vi "DeployImage_SC.vi"(8 "error in (no error)":errorcluster, 11 "SysCfgDeployRequest":T1) -> (0 "error out":errorcluster)   [LabVIEW 2016]
uses:
  <vilib>/addons/InsightCM/MessageBus/MessageLibrary/SysCfgDeployer/controls/SysCfgDeployPackageRequestBody.ctl
  <vilib>/nisyscfg/Network Settings Image.ctl
  <vilib>/nisyscfg/Set System Image (File).vi
  <vilib>/nisyscfg/Close (System).vi
  <vilib>/nisyscfg/nisyscfg.lvlib
panel:
  in  "Password":string
  in  "User Name":string="admin"
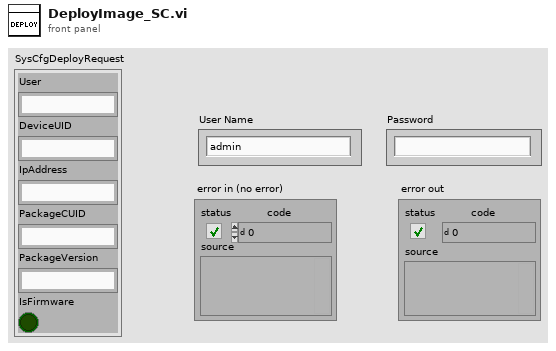
[diagram p1: front panel]
types:
  T1 = typedef "SysCfgDeployPackageRequestBody.ctl" = cluster{"User":string, "DeviceUID":string, "IpAddress":string, "PackageCUID":string, "PackageVersion":string, "IsFirmware":bool}
  T2 = typedef "nisyscfg.lvlib/Network Settings Image.ctl" = u32
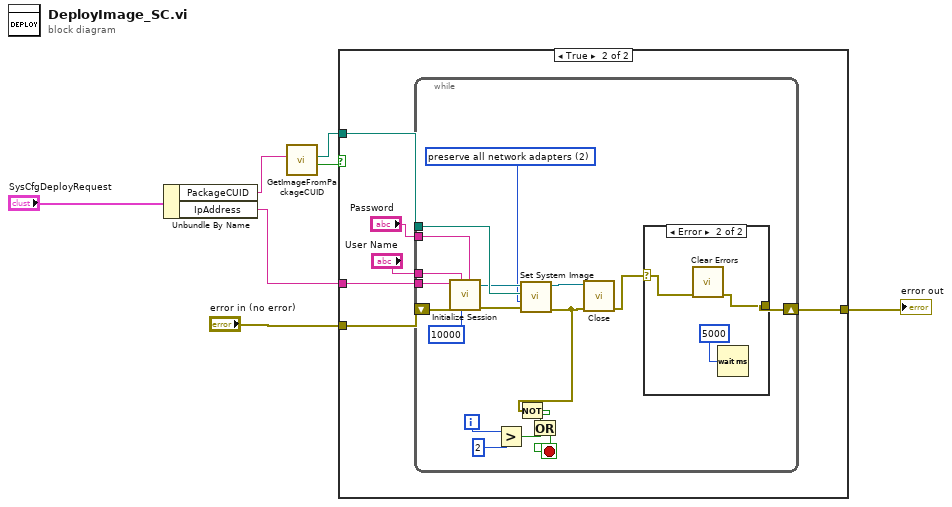
[diagram p0: block diagram]
diagram:
  n1 = Unbundle By Name("SysCfgDeployRequest") -> ("PackageCUID"=w1:string, "IpAddress"=w4:string)
  n2 = call "GetImageFromPackageCUID.vi"("PackageCUID"=w1) -> ("Found"=w2:bool, "path"=w3:path)  [unwired: 9 in]
  n3 = case shown="True" w2 {
    tunnel: "error in (no error)" -> [w8 w14]
    tunnel: [w8 w13] -> w6
    tunnel: w4 -> [_ w12]
    tunnel: w3 -> [_ w9]
    frame False {
    }
    frame True {
      n4 = while {
        tunnel: w9 -> [w32]
        shift-right: [w19] -> w13
        shift-left: w14 -> [w22]
        tunnel: "Password" -> [w24]
        tunnel: "User Name" -> [w23]
        tunnel: w12 -> [w17]
        i -> [w29]
        stop <- w31 stop-if-true
        w16 = T2 2 items=["reset all network adapters", "preserve primary, reset others", "preserve all network adapters", "preserve primary, apply others", "apply primary, reset others", "apply primary, preserve others", "apply all network adapters"] ("Network Settings (preserve primary adapter, apply others)")
        n5 = call <vilib>:"Initialize Session.vi"("Password"=w24, "Connect Timeout (4000 ms)"=u32 10000, "User Name"=w23, "error in (no error)"=w22, "Target (localhost)"=w17) -> ("error out"=w25:errorcluster, "Session out"=w21:refnum<k21>)  [unwired: 5 in]
        n6 = Greater?(x=w29, y=2) -> (0:w30:bool)
        n7 = call-poly <vilib>:"Set System Image.vi"("error in (no error)"=w25, "Network Settings (preserve primary adapter, apply others)"=w16, "Source File"=w32, "Session in"=w21) -> ("error out"=w20:errorcluster, "Session out"=w26:refnum<k21>)  [unwired: 6 in]
        n8 = Not(x=w20) -> (.not. x?=w27:bool)
        n9 = Or(x=w27, y=w30) -> (x .or. y?=w31:bool)
        n10 = call-poly <vilib>:"Close.vi"("error in (no error)"=w20, "Session in"=w26) -> ("error out"=w18:errorcluster)  [unwired: 9 in]
        n11 = case shown="Error" w18 {
          selector: w18 -> [w33 w35]
          tunnel: [w33 w34] -> w19
          frame No Error {
          }
          frame Error {
            n12 = call <vilib>:"Clear Errors.vi"("error in (no error)"=w35) -> ("error out"=w34:errorcluster)  [unwired: 5 in, 1 out]
            n13 = Wait (ms)(milliseconds to wait=u32 5000) -> ()  [unwired: 1 out]
          }
        }
      }
    }
  }
  "error out" <- w6
